vi "Ignore Hidden Files.vi"(1 "file names":path[](array[path])) -> (0 "file names 2":path[](array[path]))   [LabVIEW 2011]
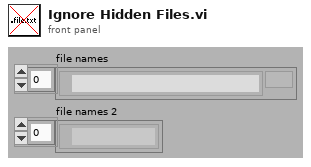
[diagram p1: front panel]
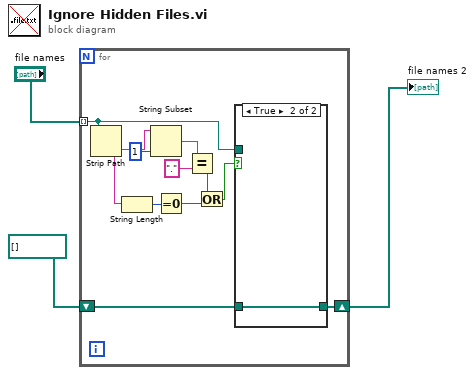
[diagram p0: block diagram]
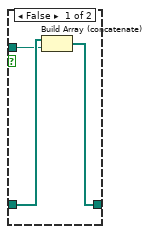
[diagram p2: hidden frame]
diagram:
  n1 = for {
    tunnel: "file names" -> [w9] mode=indexing
    shift-right: [w11] -> w2
    shift-left: path[] [] ("file names") -> [w10]
    n2 = Strip Path(path=w9) -> (name=w7:string)  [unwired: 1 out]
    n3 = String Length(string=w7) -> (length=w6:i32)
    n4 = String Subset(string=w7, length (rest)=1 ("length (rest)")) -> (substring=w12:string)  [unwired: 1 in]
    n5 = Equal To 0?(x=w6) -> (x = 0?=w5:bool)
    n6 = Equal?(x=w12, y=".") -> (x = y?=w4:bool)
    n7 = Or(x=w4, y=w5) -> (x .or. y?=w8:bool)
    n8 = case shown="True" w8 {
      tunnel: [w17 w18] -> w11
      tunnel: w10 -> [w16 w18]
      tunnel: w9 -> [w15 _]
      frame False {
        n9 = Build Array (concatenate)(w16, w15) -> (w17:path[])
      }
      frame True {
      }
    }
  }
  "file names 2" <- w2
